vi "DataHandler Start.vi"(8 "error in (no error)":errorcluster, 11 "DataProcessor in":refnum<class "DataProcessor.lvclass">) -> (0 "error out":errorcluster, 3 "DataProcessor out":refnum<class "DataProcessor.lvclass">)   [LabVIEW 2020, in "VolatusData.lvlib" / "DataProcessor.lvclass"]
uses:
  DataProcessor.lvclass
  DataProcessor.lvclass/DataProcessor.ctl
  <vilib>/ActorFramework/Actor/Actor.lvclass
  DataHandler Messages/Register Groups Msg/Register Groups Msg.lvclass
  lv-promises/Promises/Promise/Promise.lvclass
  C:/dev/lv20CE/relink/lv-volatus/Volatus/DataHandlerTask/DataHandlerTask.lvclass
  C:/dev/lv20CE/relink/lv-volatus/Volatus/Task/Task.lvclass
  C:/Program Files (x86)/National Instruments/LabVIEW 2020/vi.lib/ActorFramework/Actor/Actor.lvclass
  C:/dev/lv20CE/relink/lv-volatus/Volatus/TaskStateHandler/TaskStateHandler.lvclass
  C:/dev/lv20CE/relink/lv-volatus/Volatus/VectoMessageHandler/VectoMessageHandler.lvclass
  C:/dev/lv20CE/relink/lv-volatus/Volatus/API Provider/API Provider.lvclass
  C:/dev/lv20CE/relink/lv-volatus/Volatus/DataHandler/DataHandler.lvclass
  C:/dev/lv20CE/relink/lv-volatus/Volatus/DataProcessor/DataProcessor.lvclass
  C:/dev/lv20CE/relink/lv-volatus/Volatus/Abortable/Abortable.lvclass
  C:/dev/lv20CE/relink/lv-volatus/Volatus/Reconfigurable/Reconfigurable.lvclass
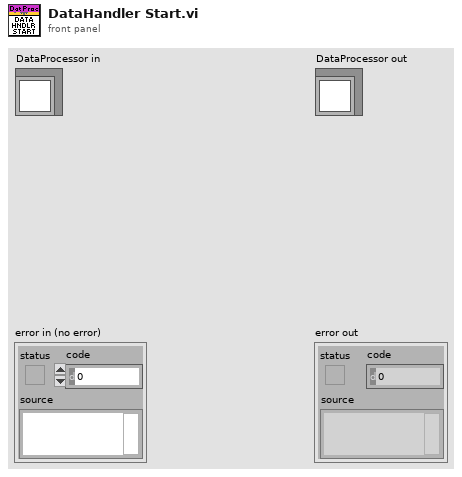
[diagram p1: front panel]
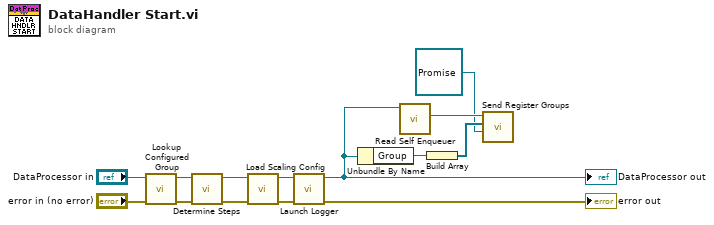
[diagram p0: block diagram]
diagram:
  n1 = call "Lookup Configured Group.vi"("error in (no error)"="error in (no error)", "DataProcessor in"="DataProcessor in") -> ("error out"=w3:errorcluster, "DataProcessor out"=w4:refnum<class "DataProcessor.lvclass">)  [unwired: 8 in]
  n2 = call "Determine Steps.vi"("error in (no error)"=w3, "DataProcessor in"=w4) -> ("error out"=w6:errorcluster, "DataProcessor out"=w5:refnum<class "DataProcessor.lvclass">)  [unwired: 8 in]
  n3 = call "Load Scaling Config.vi"("error in (no error)"=w6, "DataProcessor in"=w5) -> ("error out"=w2:errorcluster, "DataProcessor out"=w1:refnum<class "DataProcessor.lvclass">)  [unwired: 8 in]
  n4 = call "Launch Logger.vi"("error in (no error)"=w2, "DataProcessor in"=w1) -> ("error out"=→"error out":errorcluster, "DataProcessor out"=w8:refnum<class "DataProcessor.lvclass">)  [unwired: 8 in]
  "DataProcessor out" <- w8
  n5 = Unbundle By Name(w8) -> ("Group"=w10:refnum<class "Group.lvclass">)
  n6 = call <vilib>:"Read Self Enqueuer.vi"("Actor"=w8) -> ("Self Enqueuer"=w11:refnum<class "Message Enqueuer.lvclass">)  [unwired: 10 in]
  n7 = Build Array(w10) -> (w9:refnum<class "Group.lvclass">[])
  n8 = call "Send Register Groups.vi"("Promise"=refnum<class "Promise.lvclass"> refnum, "Groups"=w9, "Message Enqueuer"=w11) -> ()  [unwired: 7 in, 2 out]
